vi "Main User Event.vi"(0 "Event Data":string, 11 "Error In":errorcluster, 13 "Enum":T1) -> (4 "Message":refnum<user-event>, 15 "Error Out":errorcluster)   [LabVIEW 2020, in "I2C Controller.lvlib"]
uses:
  Typedef's/Main Event Operations.ctl
  I2C Controller.lvlib
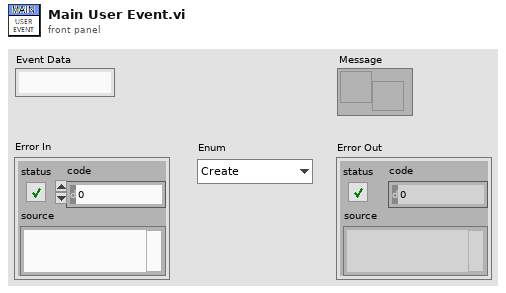
[diagram p1: front panel]
types:
  T1 = typedef "I2C Controller.lvlib/Main Event Operations.ctl" = enum16{"Create", "Generate", "Destroy"}
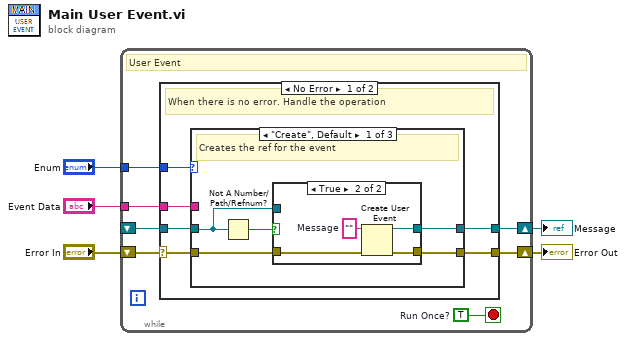
[diagram p0: block diagram]
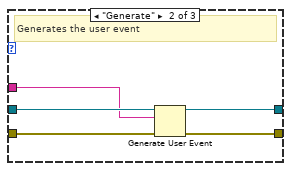
[diagram p3: hidden frame]
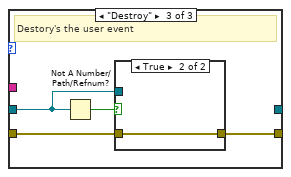
[diagram p4: hidden frame]
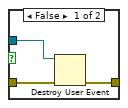
[diagram p5: hidden frame]
diagram:
  n1 = while {
    shift-right: [w10] -> w2
    shift-left: "Error In" -> [w11]
    tunnel: "Enum" -> [w9]
    shift-right: [w8] -> w1
    shift-left: _ -> [w7]
    tunnel: "Event Data" -> [w6]
    stop <- w12 stop-if-true
    w12 = TRUE  # Run Once?
    # "User Event"
    n2 = case shown="No Error" w11 {
      selector: w11 -> [w18 w44]
      tunnel: [w17 w44] -> w10
      tunnel: w9 -> [w16 _]
      tunnel: [w15 w43] -> w8
      tunnel: w7 -> [w14 w43]
      tunnel: w6 -> [w13 _]
      frame No Error {
        # "When there is no error. Handle the operation"
        n3 = case shown="\"Create\", Default" w16 {
          tunnel: w18 -> [w23 w34 w38]
          tunnel: [w22 w33 w37] -> w17
          tunnel: [w21 w31 _] -> w15
          tunnel: w14 -> [w19 w32 w35]
          tunnel: w13 -> [_ w30 _]
          frame "Create", Default {
            # "Creates the ref for the event"
            n4 = Not A Number/Path/Refnum?(number/path/refnum=w19) -> (NaN/Path/Refnum?=w20:bool)
            n5 = case shown="True" w20 {
              tunnel: w23 -> [w24 w29]
              tunnel: [w24 w28] -> w22
              tunnel: [w25 w26] -> w21
              tunnel: w19 -> [w25 _]
              frame False {
              }
              frame True {
                w27 = ""  # Message
                n6 = Create User Event(user event datatype=w27, error in=w29) -> (user event=w26:refnum<user-event>, error out=w28:errorcluster)
              }
            }
          }
          frame "Generate" {
            # "Generates the user event"
            n7 = Generate User Event(user event=w32, event data cluster=w30, error in=w34) -> (user event out=w31:refnum<user-event>, error out=w33:errorcluster)  [unwired: 1 in]
          }
          frame "Destroy" {
            # "Destory's the user event"
            n8 = Not A Number/Path/Refnum?(number/path/refnum=w35) -> (NaN/Path/Refnum?=w36:bool)
            n9 = case shown="True" w36 {
              tunnel: w38 -> [w41 w42]
              tunnel: [w40 w42] -> w37
              tunnel: w35 -> [w39 _]
              frame False {
                n10 = Destroy User Event(user event=w39, error in=w41) -> (error out=w40:errorcluster)
              }
              frame True {
              }
            }
          }
        }
      }
      frame Error {
        # "When there is error. do nothing"
      }
    }
  }
  "Error Out" <- w2
  "Message" <- w1
